vi "Unflatten From String.vi"(7 "Type and Defaults":variant, 8 "error in (no error)":errorcluster, 10 "String":string, 11 "Deserializer in":refnum<class "Deserializer.lvclass">) -> (0 "error out":errorcluster, 2 "Value":variant, 3 "Deserializer out":refnum<class "Deserializer.lvclass">)   [LabVIEW 2009, in "JKI Serialization.lvlib" / "Deserializer.lvclass"]
uses:
  Deserializer.lvclass
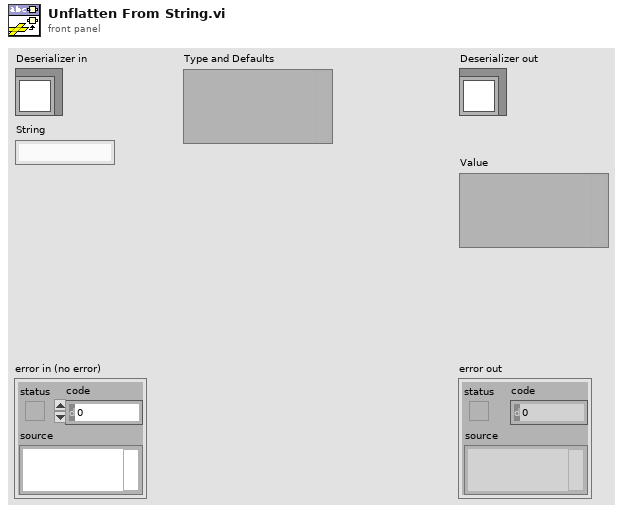
[diagram p1: front panel]
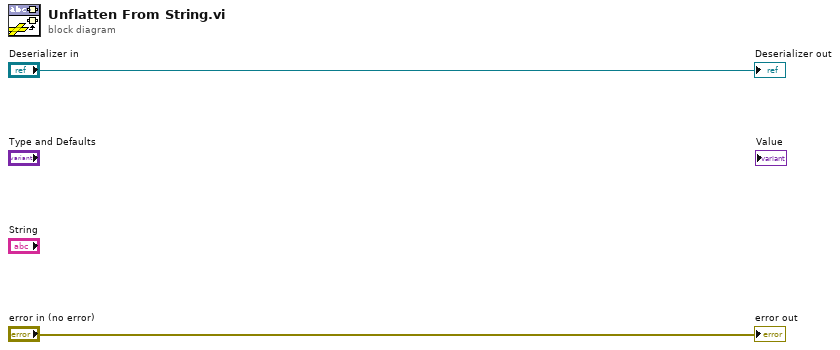
[diagram p0: block diagram]
diagram:
  "error out" <- "error in (no error)"
  "Deserializer out" <- "Deserializer in"
